vi "Reload Symbol Information Loader.vi"(8 "error in (no error)":errorcluster, 11 "TwinCAT ADS in":refnum<class "TwinCAT ADS.lvclass">) -> (0 "error out":errorcluster, 3 "TwinCAT ADS out":refnum<class "TwinCAT ADS.lvclass">)   [LabVIEW 2018, in "TwinCAT ADS.lvclass"]
uses:
  TwinCAT ADS.lvclass
  TwinCAT ADS.lvclass/TwinCAT ADS.ctl
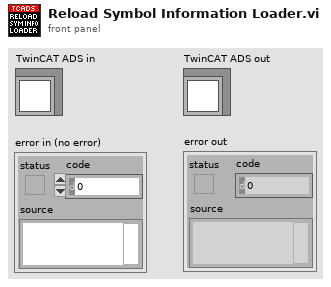
[diagram p1: front panel]
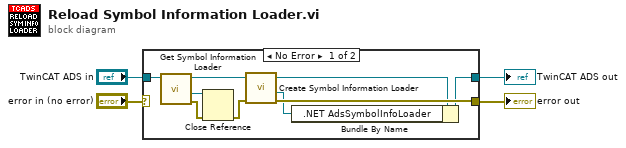
[diagram p0: block diagram]
diagram:
  n1 = case shown="No Error" "error in (no error)" {
    selector: "error in (no error)" -> [_ w15]
    tunnel: [w12 w15] -> w3
    tunnel: [w10 w14] -> w1
    tunnel: "TwinCAT ADS in" -> [w8 w14]
    frame No Error {
      n2 = call "Get Symbol Information Loader.vi"("TwinCAT ADS in"=w8) -> ("error out"=w6:errorcluster, ".NET AdsSymbolInfoLoader"=w5:refnum<k24>, "TwinCAT ADS out"=w7:refnum<class "TwinCAT ADS.lvclass">)  [unwired: 8 in]
      n3 = Close Reference(reference=w5, error in (no error)=w6) -> (error out=w13:errorcluster)
      n4 = call "Create Symbol Information Loader.vi"("error in (no error)"=w13, "TwinCAT ADS in"=w7) -> ("error out"=w12:errorcluster, "Symbol Info Loader"=w9:refnum<k24>, "TwinCAT ADS out"=w11:refnum<class "TwinCAT ADS.lvclass">)  [unwired: 7 in]
      n5 = Bundle By Name(cluster=w11, ".NET AdsSymbolInfoLoader"=w9) -> (w10:refnum<class "TwinCAT ADS.lvclass">)
    }
    frame Error {
    }
  }
  "error out" <- w3
  "TwinCAT ADS out" <- w1
